vi "Keyboard mode.vi"(11 "stop":bool) -> ()   [LabVIEW 2015]
uses:
  <vilib>/Utility/inputDevices.llb/keyboardAcquire.vi
  <vilib>/Utility/inputDevices.llb/closeKeyboard.vi
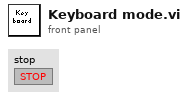
[diagram p1: front panel]
types:
  T1 = enum16{"0", "1", "2", "3", "4", "5", "6", "7", "8", "9", "A", "B", "C", "D", "E", "F", "G", "H", "I", "J", "K", "L", "M", "N", "O", "P", "Q", "R", "S", "T", "U", "V", "W", "X", "Y", "Z", "F1", "F2", "F3", "F4", "F5", "F6", "F7", "F8", "F9", "F10", "F11", "F12", "F13", "F14", "F15", "ADD", "BACK", "BACKSLASH", "CAPITAL", "COMMA", "DECIMAL", "DELETE", "DIVIDE", "DOWN", "END", "EQUALS", "ESCAPE", "GRAVE (`)", "HOME", "INSERT", "LBRACKET", "LCONTROL", "LEFT", "L ALT", "LSHIFT", "LWIN", "MINUS", "MULTIPLY", "NEXT", "NUMLOCK", "NUMPAD_0", "NUMPAD_1", "NUMPAD_2", "NUMPAD_3", "NUMPAD_4", "NUMPAD_5", "NUMPAD_6", "NUMPAD_7", "NUMPAD_8", "NUMPAD_9", "PAUSE", "PERIOD", "PRIOR (PG UP)", "RBRACKET", "RCONTROL", "RETURN", "RIGHT", "R ALT", "RSHIFT", "RWIN", "SCROLL", "SEMICOLON", "SLASH", "SPACE", "SUBTRACT", "TAB", "UP", "ENTER (num pad)", "' (quote)"}[]
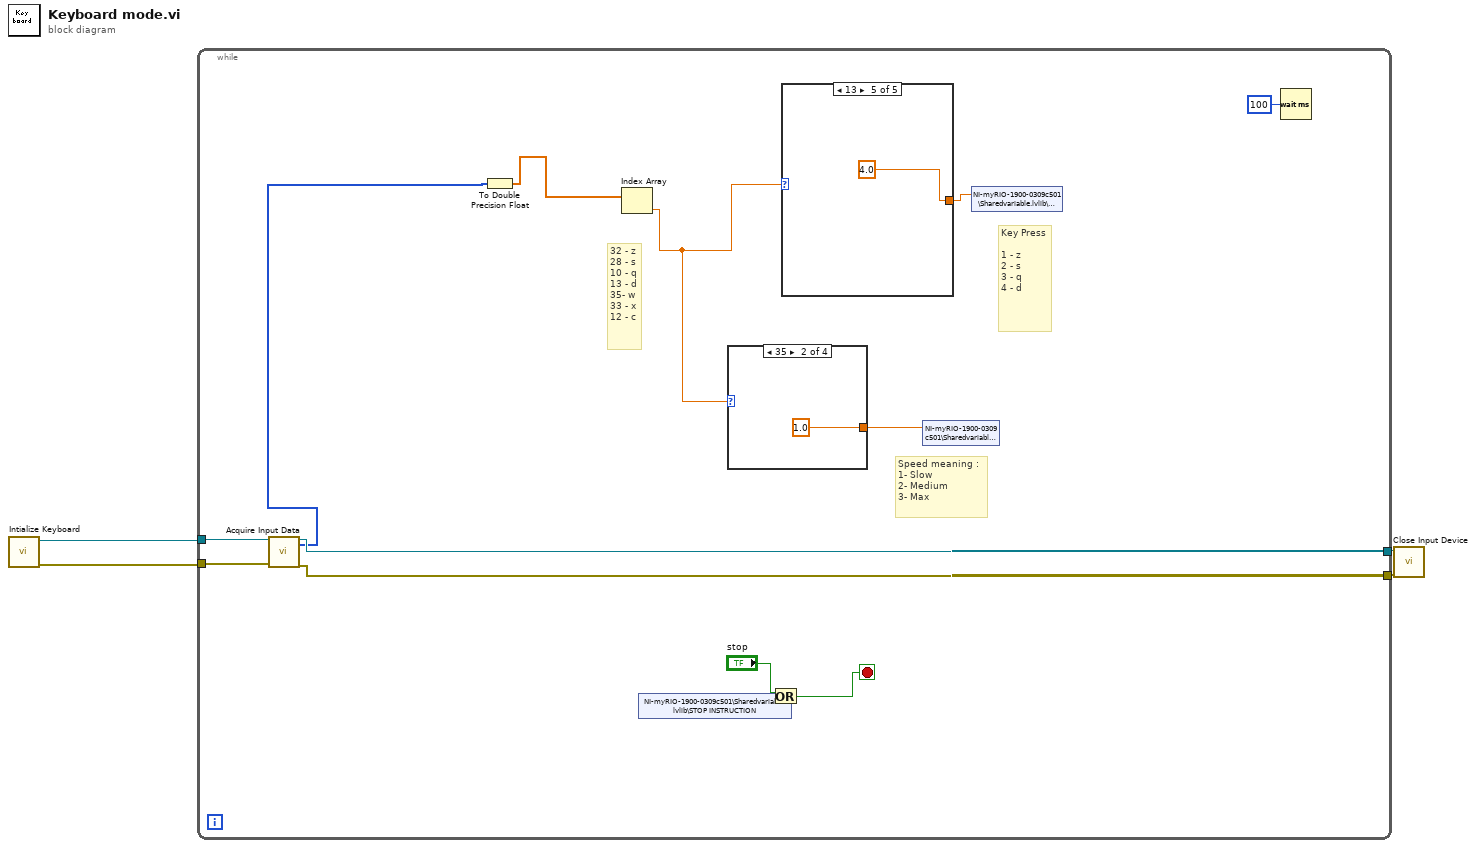
[diagram p0: block diagram]
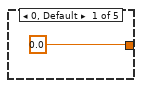
[diagram p2: hidden frame]
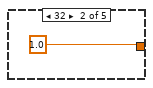
[diagram p3: hidden frame]
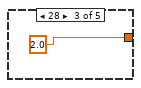
[diagram p4: hidden frame]
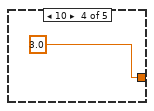
[diagram p5: hidden frame]
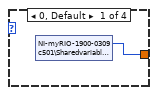
[diagram p6: hidden frame]
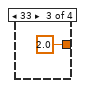
[diagram p7: hidden frame]
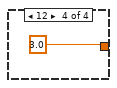
[diagram p8: hidden frame]
diagram:
  n1 = call <vilib>:"Intialize Keyboard.vi"() -> ("error out"=w3:errorcluster, "device ID"=w1:refnum<k1>)  [unwired: 10 in]
  n2 = while {
    tunnel: w1 -> [w17]
    tunnel: [w16] -> w2
    tunnel: w3 -> [w15]
    tunnel: [w14] -> w4
    stop <- w8 stop-if-true
    # "Key Press\n\n1 - z\n2 - s\n3 - q\n4 - d"
    # "Speed meaning :\n1- Slow\n2- Medium\n3- Max"
    # "32 - z\n28 - s\n10 - q\n13 - d\n35- w\n33 - x\n12 - c"
    n3 = call-poly <vilib>:"Acquire Input Data.vi"("device ID"=w17, "error in (no error)"=w15) -> ("device ID"=w16:refnum<k1>, "keys pressed"=w13:T1, "error out"=w14:errorcluster)  [unwired: 15 in]
    n4 = To Double Precision Float(number=w13) -> (double precision float=w12:dbl[])
    n5 = Index Array(array=w12) -> (element=w7:dbl)  [unwired: 1 in]
    n6 = shared-variable "NI-myRIO-1900-0309c501\\Sharedvariable.lvlib\\STOP INSTRUCTION"() -> (w9:bool)  [unwired: 1 in, 1 out]
    n7 = case shown="35" w7 {
      tunnel: [w23 1.0 2.0 3.0] -> w5
      frame 0, Default {
        n8 = shared-variable "NI-myRIO-1900-0309c501\\Sharedvariable.lvlib\\Speed"() -> (w23:u16)  [unwired: 1 in, 1 out]
      }
      frame 35 {
      }
      frame 33 {
      }
      frame 12 {
      }
    }
    n9 = Or(x="stop", y=w9) -> (x .or. y?=w8:bool)
    n10 = case shown="13" w7 {
      tunnel: [0.0 1.0 2.0 3.0 4.0] -> w6
      frame 0, Default {
      }
      frame 32 {
      }
      frame 28 {
      }
      frame 10 {
      }
      frame 13 {
      }
    }
    n11 = shared-variable "NI-myRIO-1900-0309c501\\Sharedvariable.lvlib\\Speed"(w5) -> ()  [unwired: 1 in, 1 out]
    n12 = shared-variable "NI-myRIO-1900-0309c501\\Sharedvariable.lvlib\\KeyPress"(w6) -> ()  [unwired: 1 in, 1 out]
    n13 = Wait (ms)(milliseconds to wait=u32 100) -> ()  [unwired: 1 out]
  }
  n14 = call-poly <vilib>:"Close Input Device.vi"("error in (no error)"=w4, "device ID"=w2) -> ()  [unwired: 8 in, 1 out]
